vi "set_double.vi"(8 "error in (no error)":errorcluster, 11 "ImagingModeTS090821Circular2D in":refnum<class "ImagingModeTS090821Circular2D.lvclass">) -> (0 "error out":errorcluster, 3 "ImagingModeTS090821Circular2D out":refnum<class "ImagingModeTS090821Circular2D.lvclass">)   [LabVIEW 2010, in "ImagingModeTS090821Circular2D.lvclass"]
uses:
  ImagingModeTS090821Circular2D.lvclass
  ImagingModeTS090821Circular2D.lvclass/ImagingModeTS090821Circular2D.ctl
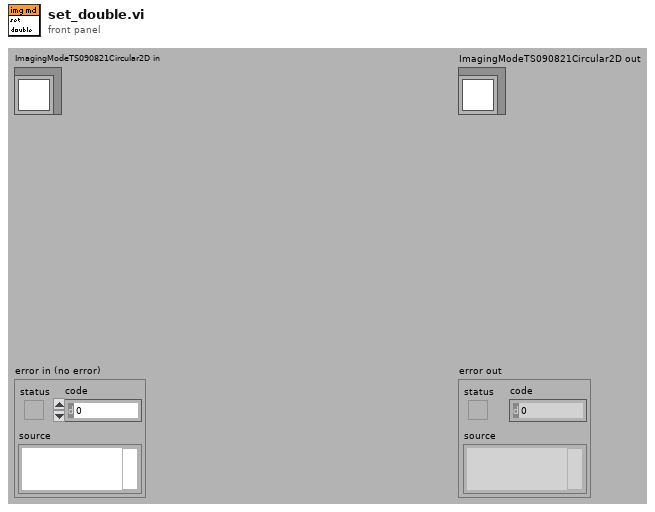
[diagram p1: front panel]
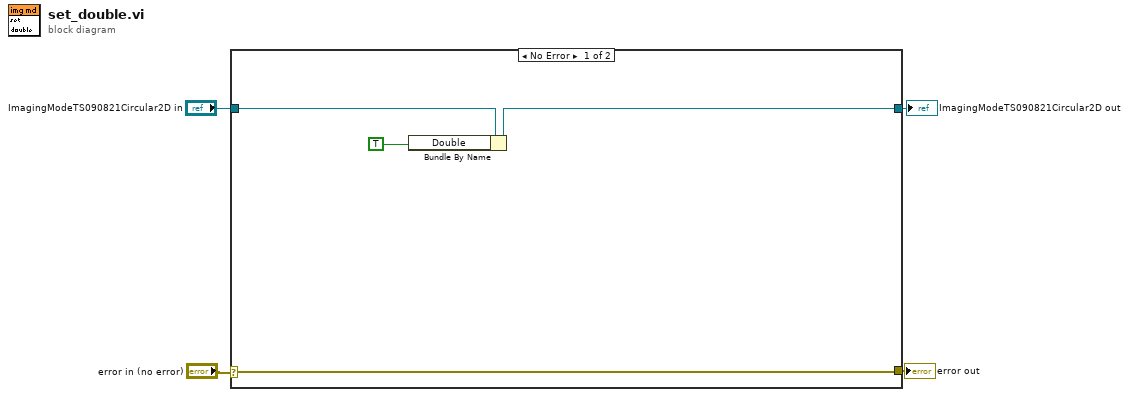
[diagram p0: block diagram]
diagram:
  n1 = case shown="No Error" "error in (no error)" {
    selector: "error in (no error)" -> [w5 w10]
    tunnel: [w5 w10] -> w3
    tunnel: [w6 w9] -> w1
    tunnel: "ImagingModeTS090821Circular2D in" -> [w8 w9]
    frame No Error {
      n2 = Bundle By Name(cluster=w8, "Double"=TRUE ("settings.Double")) -> (w6:refnum<class "ImagingModeTS090821Circular2D.lvclass">)
    }
    frame Error {
    }
  }
  "error out" <- w3
  "ImagingModeTS090821Circular2D out" <- w1
